vi "Delete All Attributes.vi"(7 "Tree ID":string, 8 "Error In":errorcluster, 11 "Tree Manager":refnum<data-value>) -> (0 "Error Out":errorcluster, 3 "Tree Manager":refnum<data-value>)   [LabVIEW 2017, in "Tree API.lvlib" / "Tree.lvclass"]
doc: "Delete all variant attributes from the Tree."
uses:
  Tree.lvclass
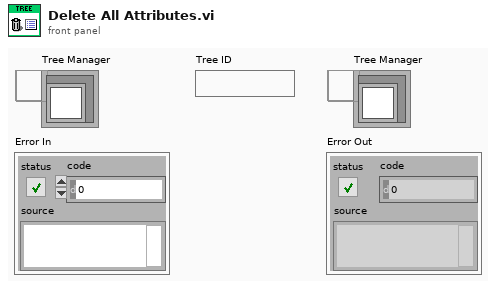
[diagram p1: front panel]
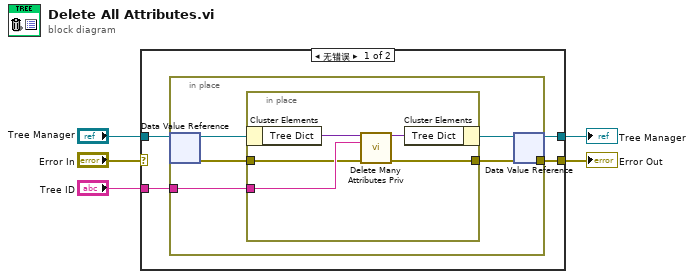
[diagram p0: block diagram]
diagram:
  n1 = case shown="无错误" "Error In" {
    selector: "Error In" -> [_ w20]
    tunnel: "Tree Manager" -> [w9 w21]
    tunnel: [w8 w21] -> w4
    tunnel: [w7 w20] -> w2
    tunnel: "Tree ID" -> [w6 _]
    frame No Error {
      n2 = in-place {
        in-place-border: [w13] -> w7
        in-place-border: w6 -> [w11]
        n3 = in-place-dvr #1(w9) -> (w14:refnum<class "Tree.lvclass">, w10:errorcluster)
        n4 = in-place {
          in-place-border: [w17] -> w13
          in-place-border: w11 -> [w18]
          in-place-border: w10 -> [w15]
          n5 = in-place-cluster #2(w14) -> ("Tree Dict"=w19:variant)
          n6 = call "Delete Many Attributes Priv.vi"("Tree Dictionary In"=w19, "Unique ID"=w18, "error in"=w15) -> ("Tree Dictionary Out"=w16:variant, "error out"=w17:errorcluster)  [unwired: 11 in]
          n7 = in-place-cluster #2("Tree Dict"=w16) -> (w12:refnum<class "Tree.lvclass">)
        }
        n8 = in-place-dvr #1(w12) -> (w8:refnum<data-value>)  [unwired: 1 out]
      }
    }
    frame Error {
    }
  }
  "Tree Manager" <- w4
  "Error Out" <- w2
